vi "setLayoutDirection.vi"(8 "Error In":errorcluster, 10 "direction":T1 items=["LeftToRight", "RightToLeft", "LayoutDirectionAuto"], 11 "LQGuiEngine In":refnum<class "LQGuiEngine.lvclass">) -> (0 "Error Out":errorcluster, 3 "LQGuiEngine Out":refnum<class "LQGuiEngine.lvclass">)   [LabVIEW 2014, in "LQGuiEngine.lvclass"]
doc: "LabVIEW-specific documentation is not yet available. See <b>https://doc.qt.io/qt-5/qguiapplication.html#setLayoutDirection</b>"
uses:
  LQGuiEngine.lvclass
  LQ Core/Qt/LayoutDirection.ctl
  LQ Core/LQIdentity/LQIdentity.lvclass/LQIdentity.ctl
  LQ Core/LQ Core.lvlib
  LQ Core/LQIdentity/LQIdentity.lvclass
  LQ Core/Qt/Qt.lvlib
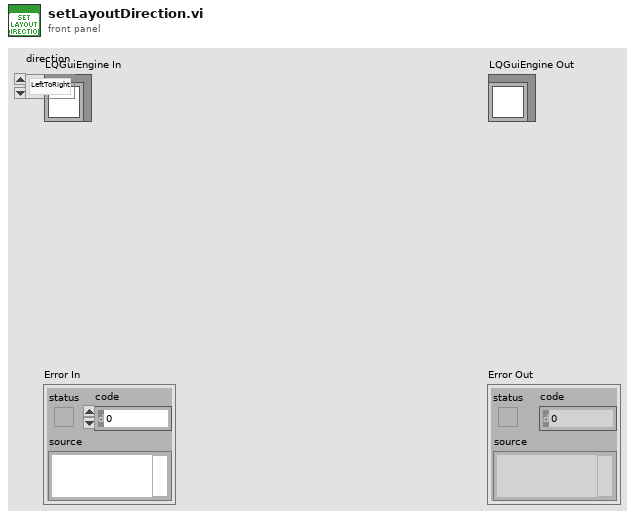
[diagram p1: front panel]
types:
  T1 = typedef "Qt.lvlib/LayoutDirection.ctl" = i32
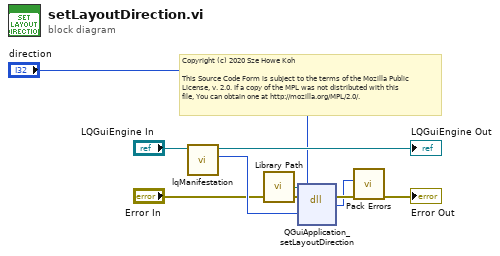
[diagram p0: block diagram]
diagram:
  # "Copyright (c) 2020 Sze Howe Koh\n\nThis Source Code Form is subject to the terms of the Mozilla Public\nLicense, v. 2.0. If a copy of the MPL was not distributed with this\nfile, You can obtain one at http://mozilla.org/MPL/2.0/."
  n1 = call "lqManifestation.vi"("LQIdentity in"="LQGuiEngine In") -> ("Manifestation"=w6:u64, "LQIdentity out"=→"LQGuiEngine Out":refnum<class "LQGuiEngine.lvclass">)  [unwired: 9 in]
  n2 = call "Library Path.vi"() -> ("Library Path"=w7:path)
  n3 = dll-call lib="?" fn="QGuiApplication_setLayoutDirection"(path in=w7, error in="Error In", "_instance"=w6, "direction"="direction") -> (error out=w4:errorcluster, w2:i32)  [unwired: 3 in, 1 out]
  n4 = call "Pack Errors.vi"("Error In"=w4, "Error Code"=w2) -> ("Error Out"=→"Error Out":errorcluster)  [unwired: 9 in]
